vi "process_watchdog.vi"() -> ()   [LabVIEW 2010]
uses:
  typedefs/control_analysis_enum.ctl
  typedefs/control_display_enum.ctl
  typedefs/control_storage_enum.ctl
  typedefs/control_daq_enum.ctl
  typedefs/data_array.ctl
  globals/exit.vi
panel:
  out "DAQ state":T1
  out "Storage state":T2
  out "Display state":T3
  out "Analysis state":T4
  out "#":i32
  out "#":i32
  out "#":i32
  out "error out":errorcluster
  out "Data_to_analysis_queue":bool
  out "Data_to_display_queue":bool
  out "Data_to_storage_queue":bool
  in  "error in (no error)":errorcluster
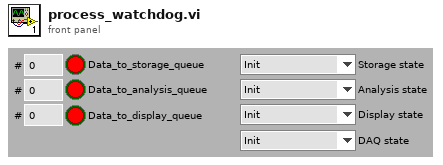
[diagram p1: front panel]
types:
  T1 = typedef "control_daq_enum.ctl" = enum16{"Init", "GetCont", "GetNoSamples", "Stop", "Quit"}
  T2 = typedef "control_storage_enum.ctl" = enum16{"Init", "Discard", "Store", "Reset", "Stop", "Quit"}
  T3 = typedef "control_display_enum.ctl" = enum16{"Init", "Display", "Quit"}
  T4 = typedef "control_analysis_enum.ctl" = enum16{"Init", "Analyze", "Reset", "Stop", "Quit"}
  T5 = typedef "data_array.ctl" = waveform(dbl)[]
  T6 = cluster{"Control DAQ Enum":T1, "variant":variant}
  T7 = cluster{"Control Analysis Enum":T4, "variant":variant}
  T8 = cluster{"Control display enum":T3, "variant":variant}
  T9 = cluster{"Control storage enum":T2, "variant":variant}
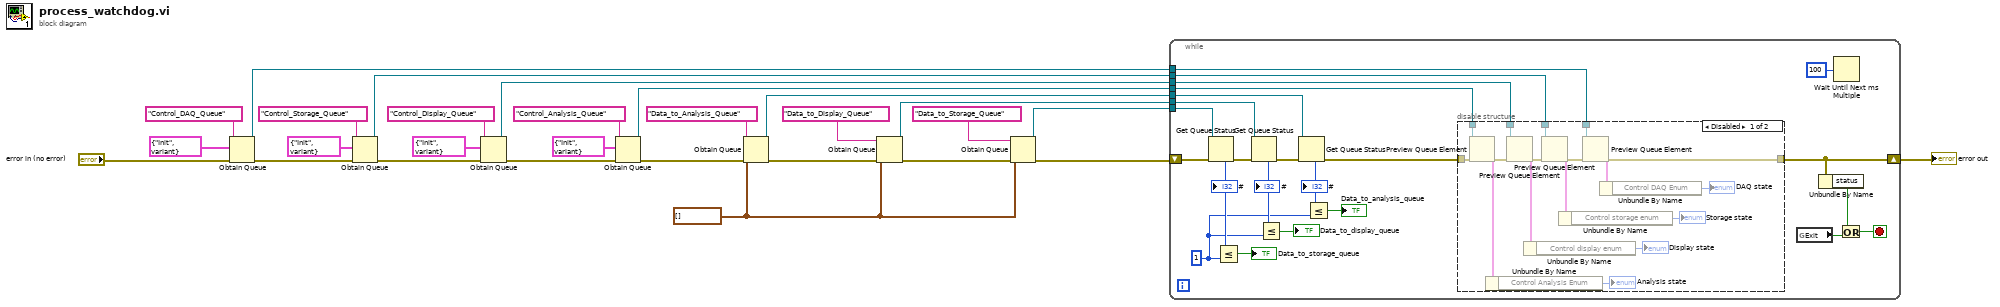
[diagram p0: block diagram]
diagram:
  w10 = T5 [] ("Data cluster")
  n1 = Obtain Queue(name (unnamed)="Control_DAQ_Queue", element data type=T6 {"Control DAQ Enum"=enum."Init", "variant"=variant} ("ControlDAQ state cluster"), error in (no error)="error in (no error)") -> (queue out=w8:refnum<queue>, error out=w25:errorcluster)  [unwired: 2 in, 1 out]
  n2 = Obtain Queue(name (unnamed)="Control_Storage_Queue", element data type=T9 {"Control storage enum"=enum."Init", "variant"=variant}, error in (no error)=w25) -> (queue out=w7:refnum<queue>, error out=w24:errorcluster)  [unwired: 2 in, 1 out]
  n3 = Obtain Queue(name (unnamed)="Control_Display_Queue", element data type=T8 {"Control display enum"=enum."Init", "variant"=variant}, error in (no error)=w24) -> (queue out=w6:refnum<queue>, error out=w21:errorcluster)  [unwired: 2 in, 1 out]
  n4 = Obtain Queue(name (unnamed)="Control_Analysis_Queue", element data type=T7 {"Control Analysis Enum"=enum."Init", "variant"=variant}, error in (no error)=w21) -> (queue out=w5:refnum<queue>, error out=w15:errorcluster)  [unwired: 2 in, 1 out]
  n5 = Obtain Queue(name (unnamed)="Data_to_Analysis_Queue", element data type=w10, error in (no error)=w15) -> (queue out=w4:refnum<queue>, error out=w12:errorcluster)  [unwired: 2 in, 1 out]
  n6 = Obtain Queue(name (unnamed)="Data_to_Display_Queue", element data type=w10, error in (no error)=w12) -> (queue out=w3:refnum<queue>, error out=w14:errorcluster)  [unwired: 2 in, 1 out]
  n7 = Obtain Queue(name (unnamed)="Data_to_Storage_Queue", element data type=w10, error in (no error)=w14) -> (queue out=w2:refnum<queue>, error out=w9:errorcluster)  [unwired: 2 in, 1 out]
  n8 = while {
    tunnel: w8 -> [w30]
    tunnel: w7 -> [w31]
    tunnel: w6 -> [w32]
    tunnel: w5 -> [w33]
    tunnel: w4 -> [w42]
    tunnel: w3 -> [w46]
    tunnel: w2 -> [w50]
    shift-right: [w29] -> w1
    shift-left: w9 -> [w51]
    stop <- w36 stop-if-true
    w39 = 1 ("y")
    n9 = Get Queue Status(queue=w50, error in (no error)=w51) -> (error out=w47:errorcluster, # elements in queue=w49:i32)  [unwired: 1 in, 6 out]
    "#" <- w49
    n10 = Less Or Equal?(x=w49, y=w39) -> (x <= y?=→"Data_to_storage_queue":bool)
    n11 = Get Queue Status(queue=w46, error in (no error)=w47) -> (error out=w43:errorcluster, # elements in queue=w44:i32)  [unwired: 1 in, 6 out]
    "#" <- w44
    n12 = Less Or Equal?(x=w44, y=w39) -> (x <= y?=→"Data_to_display_queue":bool)
    n13 = Get Queue Status(queue=w42, error in (no error)=w43) -> (error out=w34:errorcluster, # elements in queue=w40:i32)  [unwired: 1 in, 6 out]
    "#" <- w40
    n14 = Less Or Equal?(x=w40, y=w39) -> (x <= y?=→"Data_to_analysis_queue":bool)
    n15 = disable-structure shown="Disabled" {
      disable-tunnel: w34 -> [w68 _]
      disable-tunnel: w33 -> [w67 _]
      disable-tunnel: w32 -> [w63 _]
      disable-tunnel: w31 -> [w59 _]
      disable-tunnel: w30 -> [w56 _]
      disable-tunnel: [w54 _] -> w29
      frame Disabled {
        n16 = Preview Queue Element(queue=w67, error in (no error)=w68) -> (element=w66:T7, error out=w64:errorcluster)  [unwired: 1 in, 2 out]
        n17 = Unbundle By Name(w66) -> ("Control Analysis Enum"=→"Analysis state":T4)
        n18 = Preview Queue Element(queue=w63, error in (no error)=w64) -> (element=w62:T8, error out=w60:errorcluster)  [unwired: 1 in, 2 out]
        n19 = Unbundle By Name(w62) -> ("Control display enum"=→"Display state":T3)
        n20 = Preview Queue Element(queue=w59, error in (no error)=w60) -> (element=w58:T9, error out=w55:errorcluster)  [unwired: 1 in, 2 out]
        n21 = Unbundle By Name(w58) -> ("Control storage enum"=→"Storage state":T2)
        n22 = Preview Queue Element(queue=w56, error in (no error)=w55) -> (element=w53:T6, error out=w54:errorcluster)  [unwired: 1 in, 2 out]
        n23 = Unbundle By Name(w53) -> ("Control DAQ Enum"=→"DAQ state":T1)
      }
      frame Enabled {
      }
    }
    n24 = global read "exit.vi" "Exit"() -> (w35:bool)
    n25 = Unbundle By Name(w29) -> ("status"=w37:bool)
    n26 = Wait Until Next ms Multiple(millisecond multiple=u32 100) -> ()  [unwired: 1 out]
    n27 = Or(x=w37, y=w35) -> (x .or. y?=w36:bool)
  }
  "error out" <- w1
